vi "Rating.vi"(10 "Class Predict":dbl[](array[numeric]), 11 "Class Real":dbl[](array[numeric])) -> (2 "Bad":i32, 3 "Good":i32)   [LabVIEW 2020]
doc: "Defines the number of good and bad predictions"
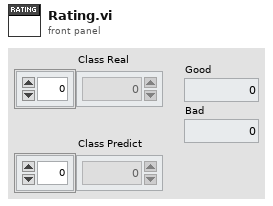
[diagram p1: front panel]
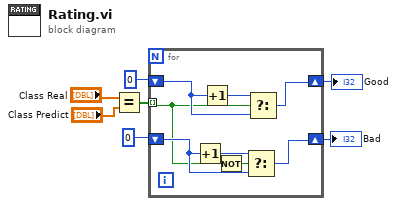
[diagram p0: block diagram]
diagram:
  n1 = Equal?(x="Class Real", y="Class Predict") -> (x = y?=w5:bool[])
  n2 = for {
    tunnel: w5 -> [w9] mode=indexing
    shift-right: [w14] -> w2
    shift-left: 0 -> [w15]
    shift-right: [w11] -> w1
    shift-left: 0 -> [w10]
    n3 = Increment(x=w10) -> (x+1=w12:i32)
    n4 = Increment(x=w15) -> (x+1=w13:i32)
    n5 = Not(x=w9) -> (.not. x?=w8:bool)
    n6 = Select(t=w12, s=w8, f=w10) -> (s? t:f=w11:i32)
    n7 = Select(t=w13, s=w9, f=w15) -> (s? t:f=w14:i32)
  }
  "Bad" <- w1
  "Good" <- w2
